vi "SaveSubVi.vi"(0 "UDP message":string, 1 "command":string="setSave", 7 "variables":string[][](array[string]), 9 "Arguments":string, 11 "error in":errorcluster) -> (4 "UDP message out":string, 8 "variables out":string[][](array[string]), 10 "new Value":string, 15 "error out":errorcluster)   [LabVIEW 2009]
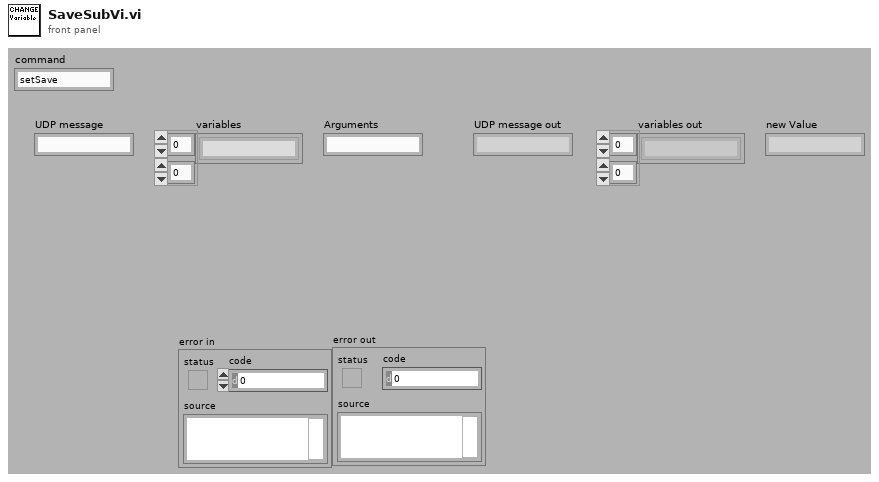
[diagram p1: front panel]
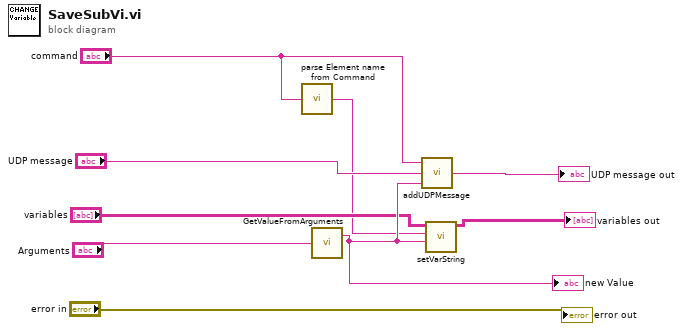
[diagram p0: block diagram]
diagram:
  n1 = call "parse Element name from Command.vi"("setcommand"="command") -> ("element name"=w2:string)
  n2 = call "GetValueFromArguments.vi"("Arguments"="Arguments") -> ("setValue"=w9:string)  [unwired: 1 out]
  "new Value" <- w9
  n3 = call "addUDPMessage.vi"("value"=w9, "UDP message"="UDP message", "command"="command") -> ("UDP message out"=→"UDP message out":string)
  n4 = call "setVarString.vi"("value"=w9, "element"=w2, "variables"="variables") -> ("variables out"=→"variables out":string[][])  [unwired: 8 in]
  "error out" <- "error in"
